vi "Init SUT.vi"(8 "error in (no error)":errorcluster, 11 "Text Report Test in":refnum<class "Text Report Test.lvclass">) -> (0 "error out":errorcluster, 3 "Text Report out":refnum<class "Text Report.lvclass">)   [LabVIEW 2020, in "Text Report Test.lvclass"]
uses:
  Text Report Test.lvclass
  Text Report Test.lvclass/Text Report Test.ctl
  source/Plugins/Text Report/Text Report.lvclass
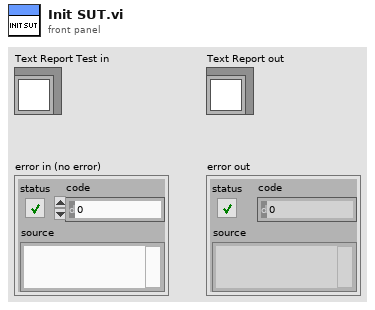
[diagram p1: front panel]
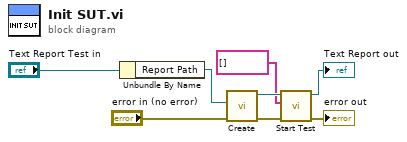
[diagram p0: block diagram]
diagram:
  n1 = Unbundle By Name("Text Report Test in") -> ("Report Path"=w8:path)
  n2 = call "Create.vi"("error in (no error)"="error in (no error)", "Report Path"=w8) -> ("error out"=w6:errorcluster, "Text Report"=w7:refnum<class "Text Report.lvclass">)  [unwired: 8 in]
  n3 = call-dynamic "Start Test.vi"("error in (no error)"=w6, "Tests"=string[] [], "Text Report In"=w7) -> ("error out"=→"error out":errorcluster, "Text Report Out"=→"Text Report out":refnum<class "Text Report.lvclass">)  [unwired: 7 in]
